vi "TIO RPC Form Request.vi"(10 "Payload":string, 11 "Topic":string="dev.name") -> (2 "Request ID":u16=60741 format="%04x", 3 "String out":string)   [LabVIEW 2022 SP3]
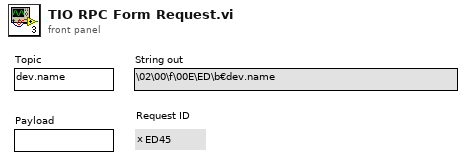
[diagram p1: front panel]
types:
  T1 = enum16{"big-endian, network order", "native, host order", "little-endian"}
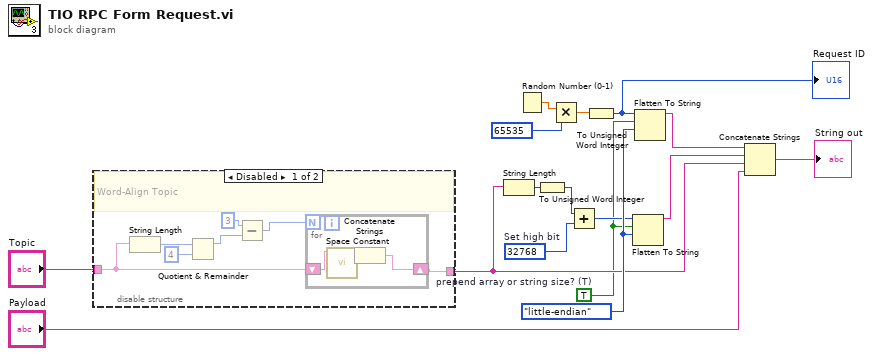
[diagram p0: block diagram]
diagram:
  w2 = TRUE  # prepend array or string size? (T)
  w11 = u16 32768  # Set high bit
  w14 = T1."little-endian" ("byte order (0:big-endian, network order)")
  n1 = disable-structure shown="Disabled" {
    disable-tunnel: "Topic" -> [w18 w27]
    disable-tunnel: [w17 w27] -> w3
    frame Disabled {
      # "Word-Align Topic"
      n2 = String Length(string=w18) -> (length=w22:i32)
      n3 = Quotient & Remainder(x=w22, y=4) -> (x-y*floor(x/y)=w21:i32)  [unwired: 1 out]
      n4 = Subtract(x=3, y=w21) -> (x-y=w19:i32)
      n5 = for {
        N: w19 -> [_]
        shift-right: [w25] -> w17
        shift-left: w18 -> [w26]
        n6 = call <vilib>:"Space Constant.vi"() -> ("String"=w24:string)
        n7 = Concatenate Strings(w26, w24) -> (w25:string)
      }
    }
    frame Enabled {
    }
  }
  n8 = String Length(string=w3) -> (length=w10:i32)
  n9 = Random Number (0-1)() -> (number: 0 to 1=w7:dbl)
  n10 = To Unsigned Word Integer(number=w10) -> (unsigned 16bit integer=w12:u16)
  n11 = Multiply(x=w7, y=u16 65535) -> (x*y=w9:dbl)
  n12 = Add(x=w12, y=w11) -> (x+y=w13:u16)
  n13 = To Unsigned Word Integer(number=w9) -> (unsigned 16bit integer=w6:u16)
  "Request ID" <- w6
  n14 = Flatten To String(anything=w13, prepend array or string size? (T)=w2, byte order (0:big-endian, network order)=w14) -> (data string=w16:string)  [unwired: 1 in, 2 out]
  n15 = Flatten To String(anything=w6, prepend array or string size? (T)=w2, byte order (0:big-endian, network order)=w14) -> (data string=w15:string)  [unwired: 1 in, 2 out]
  n16 = Concatenate Strings(w15, w16, w3, "Payload") -> (→"String out":string)
